vi "Delete Old Library from Disk.vi"(8 "error in (no error)":errorcluster, 10 "folder to delete":string) -> (0 "error out":errorcluster)   [LabVIEW 2020]
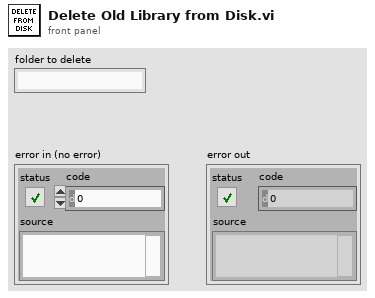
[diagram p1: front panel]
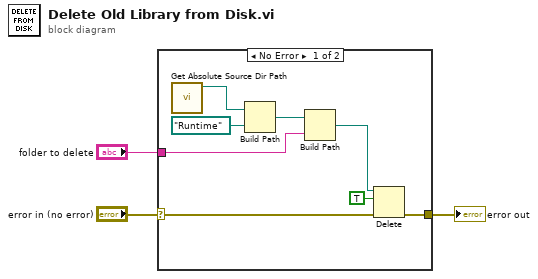
[diagram p0: block diagram]
diagram:
  n1 = case shown="No Error" "error in (no error)" {
    selector: "error in (no error)" -> [w9 w12]
    tunnel: "folder to delete" -> [w10 _]
    tunnel: [w6 w12] -> w1
    frame No Error {
      n2 = call "Get Absolute Source Dir Path.vi"() -> ("source dir"=w5:path)  [unwired: 11 in]
      n3 = Build Path(base path=w5, name or relative path=path "Runtime") -> (appended path=w11:path)
      n4 = Build Path(base path=w11, name or relative path=w10) -> (appended path=w8:path)
      n5 = Delete(path (use dialog)=w8, entire hierarchy (F)=TRUE, error in=w9) -> (error out=w6:errorcluster)  [unwired: 2 in, 2 out]
    }
    frame Error {
    }
  }
  "error out" <- w1
